vi "test_Compare Avg Access Speed - Var Dict.vi"() -> ()   [LabVIEW 2015]
uses:
  Test Object/Test Object.lvclass
  Test Object/Test Object.lvclass/Test Object.ctl
  objdict/objdict.lvclass
panel:
  out "Average test duration [ms]":dbl[][](array[numeric]) format="%#.6p"
  # "Access Object"
  # "Access and Read Object"
  # "Access and Modify Object"
  # "Variant dict"
  # "objdict"
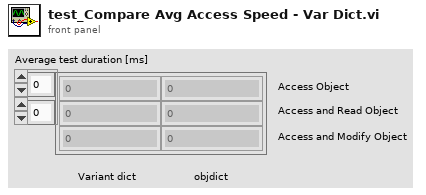
[diagram p1: front panel]
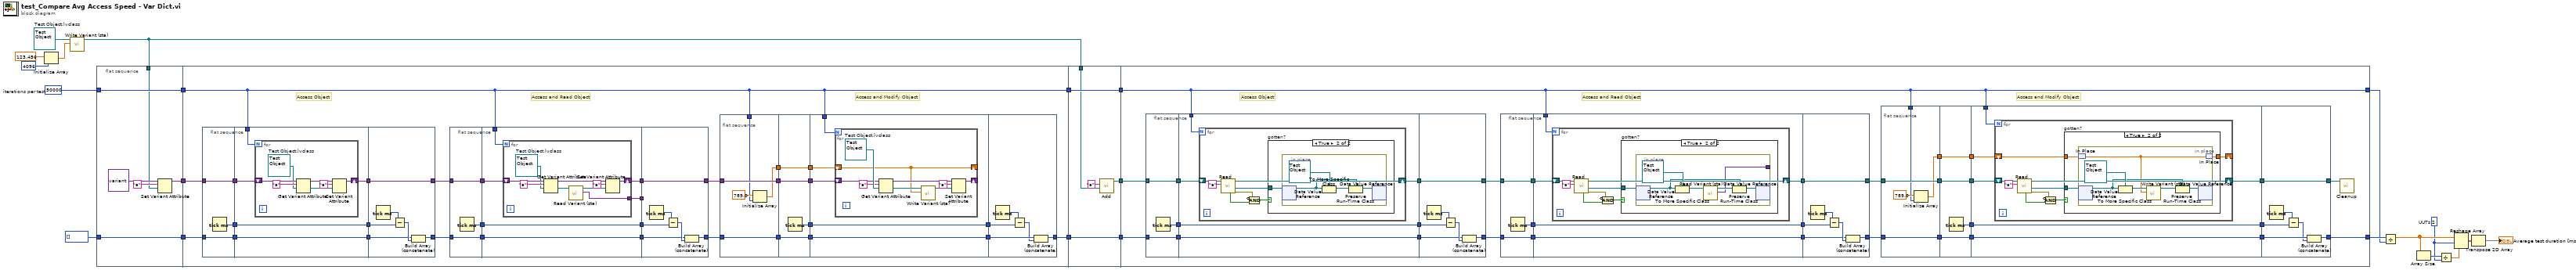
[diagram p0: block diagram]
diagram:
  w2 = 2  # UUTs
  w18 = 50000  # iterations per test
  w23 = refnum<class "Test Object.lvclass"> refnum  # Test Object.lvclass
  n1 = Initialize Array(123.456, 4096) -> (w20:dbl[])
  n2 = call "Write Variant (sta).vi"("Variant"=w20, "Test Object in"=w23) -> ("Test Object out"=w8:refnum<class "Test Object.lvclass">)  [unwired: 9 in]
  n3 = flat-sequence {
    tunnel: w18 -> [w28]
    tunnel: u32[] [] -> [w29]
    tunnel: [w29] -> w13
    tunnel: [w28] -> w12
    tunnel: w8 -> [w25]
    tunnel: [w24] -> w11
    tunnel: w13 -> [w53]
    tunnel: w12 -> [w30]
    tunnel: w11 -> [w42]
    tunnel: [w44] -> w10
    tunnel: [w30] -> w9
    tunnel: w10 -> [w137]
    tunnel: w9 -> [w136]
    tunnel: w8 -> [w135]
    tunnel: [w137] -> w7
    tunnel: [w136] -> w6
    tunnel: [w133] -> w5
    tunnel: [w140] -> w15
    tunnel: [w141] -> w16
    tunnel: w7 -> [w142]
    tunnel: w6 -> [w140]
    tunnel: w5 -> [w143]
    frame #0 {
      n4 = Set Variant Attribute(Variant=variant, name="a", value=w25) -> (Variant out=w24:variant)  [unwired: 1 in, 2 out]
    }
    frame #1 {
      # "Access and Read Object"
      # "Access and Modify Object"
      # "Access Object"
      n5 = flat-sequence {
        tunnel: w42 -> [w114]
        tunnel: [w114] -> w59
        tunnel: [w113] -> w58
        tunnel: w53 -> [w112]
        tunnel: [w112] -> w52
        tunnel: w59 -> [w119]
        tunnel: w58 -> [w118]
        tunnel: [w118] -> w57
        tunnel: w52 -> [w117]
        tunnel: [w117] -> w51
        tunnel: w30 -> [w116]
        tunnel: [w115] -> w43
        tunnel: w57 -> [w132]
        tunnel: w51 -> [w129]
        tunnel: [w128] -> w33
        tunnel: [w127] -> w34
        tunnel: w43 -> [w127]
        frame #0 {
          n6 = Tick Count (ms)() -> (millisecond timer value=w113:u32)
        }
        frame #1 {
          n7 = for {
            N: w116 -> [_]
            shift-right: [w124] -> w115
            shift-left: w119 -> [w126]
            w120 = refnum<class "Test Object.lvclass"> refnum  # Test Object.lvclass
            n8 = Get Variant Attribute(Variant=w126, name="a", default value (empty Variant)=w120) -> (duplicate Variant=w125:variant, value=w122:refnum<class "Test Object.lvclass">)  [unwired: 1 in, 2 out]
            n9 = Set Variant Attribute(Variant=w125, name="a", value=w122) -> (Variant out=w124:variant)  [unwired: 1 in, 2 out]
          }
        }
        frame #2 {
          n10 = Tick Count (ms)() -> (millisecond timer value=w131:u32)
          n11 = Subtract(x=w131, y=w132) -> (x-y=w130:u32)
          n12 = Build Array (concatenate)(w129, w130) -> (w128:u32[])
        }
      }
      n13 = flat-sequence {
        tunnel: w34 -> [w62]
        tunnel: [w62] -> w41
        tunnel: [w61] -> w40
        tunnel: w33 -> [w60]
        tunnel: [w60] -> w39
        tunnel: w41 -> [w68]
        tunnel: w40 -> [w67]
        tunnel: [w67] -> w38
        tunnel: w39 -> [w66]
        tunnel: [w66] -> w37
        tunnel: w30 -> [w65]
        tunnel: [w64] -> w36
        tunnel: [w63] -> w35
        tunnel: w38 -> [w83]
        tunnel: w37 -> [w80]
        tunnel: [w79] -> w31
        tunnel: [w78] -> w32
        tunnel: w36 -> [w78]
        tunnel: w35 -> [_]
        frame #0 {
          n14 = Tick Count (ms)() -> (millisecond timer value=w61:u32)
        }
        frame #1 {
          n15 = for {
            N: w65 -> [_]
            shift-right: [w75] -> w64
            shift-left: w68 -> [w77]
            tunnel: [w69] -> w63
            w71 = refnum<class "Test Object.lvclass"> refnum  # Test Object.lvclass
            n16 = Get Variant Attribute(Variant=w77, name="a", default value (empty Variant)=w71) -> (duplicate Variant=w76:variant, value=w73:refnum<class "Test Object.lvclass">)  [unwired: 1 in, 2 out]
            n17 = call "Read Variant (sta).vi"("Test Object in"=w73) -> ("Variant"=w69:variant, "Test Object out"=w70:refnum<class "Test Object.lvclass">)  [unwired: 9 in]
            n18 = Set Variant Attribute(Variant=w76, name="a", value=w70) -> (Variant out=w75:variant)  [unwired: 1 in, 2 out]
          }
        }
        frame #2 {
          n19 = Tick Count (ms)() -> (millisecond timer value=w82:u32)
          n20 = Subtract(x=w82, y=w83) -> (x-y=w81:u32)
          n21 = Build Array (concatenate)(w80, w81) -> (w79:u32[])
        }
      }
      n22 = flat-sequence {
        tunnel: w31 -> [w87]
        tunnel: w32 -> [w88]
        tunnel: [w88] -> w48
        tunnel: [w87] -> w47
        tunnel: [w85] -> w45
        tunnel: w30 -> [w84]
        tunnel: [w92] -> w56
        tunnel: [w91] -> w55
        tunnel: [w90] -> w50
        tunnel: w48 -> [w92]
        tunnel: w47 -> [w90]
        tunnel: [w89] -> w46
        tunnel: w45 -> [w89]
        tunnel: w56 -> [w97]
        tunnel: w55 -> [w96]
        tunnel: [w96] -> w54
        tunnel: w50 -> [w95]
        tunnel: [w95] -> w49
        tunnel: w30 -> [w94]
        tunnel: w46 -> [w93]
        tunnel: w54 -> [w111]
        tunnel: w49 -> [w109]
        tunnel: [w107] -> w44
        frame #0 {
          n23 = Initialize Array(789.0, w84) -> (w85:dbl[])
        }
        frame #1 {
          n24 = Tick Count (ms)() -> (millisecond timer value=w91:u32)
        }
        frame #2 {
          n25 = for {
            N: w94 -> [_]
            shift-right: [w100] -> _
            shift-left: w97 -> [w101]
            shift-right: [w98] -> _
            shift-left: w93 -> [w98]
            w106 = refnum<class "Test Object.lvclass"> refnum  # Test Object.lvclass
            n26 = Get Variant Attribute(Variant=w101, name="a", default value (empty Variant)=w106) -> (duplicate Variant=w102:variant, value=w105:refnum<class "Test Object.lvclass">)  [unwired: 1 in, 2 out]
            n27 = call "Write Variant (sta).vi"("Variant"=w98, "Test Object in"=w105) -> ("Test Object out"=w99:refnum<class "Test Object.lvclass">)  [unwired: 9 in]
            n28 = Set Variant Attribute(Variant=w102, name="a", value=w99) -> (Variant out=w100:variant)  [unwired: 1 in, 2 out]
          }
        }
        frame #3 {
          n29 = Tick Count (ms)() -> (millisecond timer value=w110:u32)
          n30 = Subtract(x=w110, y=w111) -> (x-y=w108:u32)
          n31 = Build Array (concatenate)(w109, w108) -> (w107:u32[])
        }
      }
    }
    frame #2 {
      n32 = call "Add.vi"("LabVIEW Object"=w135, "key"="a") -> ("Object Dictionary out"=w133:refnum<class "objdict.lvclass">)  [unwired: 8 in, 1 out]
    }
    frame #3 {
      # "Access and Read Object"
      # "Access and Modify Object"
      # "Access Object"
      n33 = flat-sequence {
        tunnel: w143 -> [w239]
        tunnel: [w239] -> w168
        tunnel: [w238] -> w167
        tunnel: w142 -> [w237]
        tunnel: [w237] -> w166
        tunnel: w168 -> [w244]
        tunnel: w167 -> [w243]
        tunnel: [w243] -> w165
        tunnel: w166 -> [w242]
        tunnel: [w242] -> w164
        tunnel: w140 -> [w241]
        tunnel: [w240] -> w163
        tunnel: w165 -> [w262]
        tunnel: w164 -> [w259]
        tunnel: [w258] -> w146
        tunnel: [w257] -> w147
        tunnel: w163 -> [w257]
        frame #0 {
          n34 = Tick Count (ms)() -> (millisecond timer value=w238:u32)
        }
        frame #1 {
          n35 = for {
            N: w241 -> [_]
            shift-right: [w246] -> w240
            shift-left: w244 -> [w251]
            n36 = call "Read.vi"("key"="a", "Object Dictionary in"=w251) -> ("error out"=w247:errorcluster, "Object ref"=w248:refnum<data-value>, "Object Dictionary out"=w246:refnum<class "objdict.lvclass">, "found"=w245:bool)  [unwired: 6 in]
            n37 = Compound Arithmetic op=AND(invert w247, w245) -> (w249:bool)
            n38 = case "gotten?" shown="True" w249 {
              tunnel: w248 -> [_ w252]
              frame False {
              }
              frame True {
                n39 = in-place {
                  n40 = in-place-dvr #1(w252) -> (w255:refnum<class>)  [unwired: 1 out]
                  n41 = To More Specific Class(target class=refnum<class "Test Object.lvclass"> refnum ("Test Object.lvclass"), reference=w255) -> (specific class reference=w253:refnum<class "Test Object.lvclass">)  [unwired: 1 in, 1 out]
                  n42 = Preserve Run-Time Class(object in=w253, 2:w255) -> (object out=w254:refnum<class>)  [unwired: 1 in, 1 out]
                  n43 = in-place-dvr #1(w254) -> ()  [unwired: 2 out]
                }
              }
            }
          }
        }
        frame #2 {
          n44 = Tick Count (ms)() -> (millisecond timer value=w261:u32)
          n45 = Subtract(x=w261, y=w262) -> (x-y=w260:u32)
          n46 = Build Array (concatenate)(w259, w260) -> (w258:u32[])
        }
      }
      n47 = flat-sequence {
        tunnel: w147 -> [w171]
        tunnel: [w171] -> w153
        tunnel: [w170] -> w152
        tunnel: w146 -> [w169]
        tunnel: [w169] -> w151
        tunnel: w153 -> [w174]
        tunnel: w152 -> [w176]
        tunnel: [w176] -> w150
        tunnel: w151 -> [w175]
        tunnel: [w175] -> w149
        tunnel: w140 -> [w173]
        tunnel: [w172] -> w148
        tunnel: w150 -> [w196]
        tunnel: w149 -> [w193]
        tunnel: [w192] -> w144
        tunnel: [w191] -> w145
        tunnel: w148 -> [w191]
        frame #0 {
          n48 = Tick Count (ms)() -> (millisecond timer value=w170:u32)
        }
        frame #1 {
          n49 = for {
            N: w173 -> [_]
            shift-right: [w178] -> w172
            shift-left: w174 -> [w183]
            n50 = call "Read.vi"("key"="a", "Object Dictionary in"=w183) -> ("error out"=w179:errorcluster, "Object ref"=w180:refnum<data-value>, "Object Dictionary out"=w178:refnum<class "objdict.lvclass">, "found"=w177:bool)  [unwired: 6 in]
            n51 = Compound Arithmetic op=AND(invert w179, w177) -> (w181:bool)
            n52 = case "gotten?" shown="True" w181 {
              tunnel: w180 -> [_ w184]
              frame False {
              }
              frame True {
                n53 = in-place {
                  in-place-border: [w185] -> _
                  n54 = in-place-dvr #2(w184) -> (w189:refnum<class>)  [unwired: 1 out]
                  n55 = To More Specific Class(target class=refnum<class "Test Object.lvclass"> refnum ("Test Object.lvclass"), reference=w189) -> (specific class reference=w187:refnum<class "Test Object.lvclass">)  [unwired: 1 in, 1 out]
                  n56 = call "Read Variant (sta).vi"("Test Object in"=w187) -> ("Variant"=w185:variant, "Test Object out"=w186:refnum<class "Test Object.lvclass">)  [unwired: 9 in]
                  n57 = Preserve Run-Time Class(object in=w186, 2:w189) -> (object out=w188:refnum<class>)  [unwired: 1 in, 1 out]
                  n58 = in-place-dvr #2(w188) -> ()  [unwired: 2 out]
                }
              }
            }
          }
        }
        frame #2 {
          n59 = Tick Count (ms)() -> (millisecond timer value=w195:u32)
          n60 = Subtract(x=w195, y=w196) -> (x-y=w194:u32)
          n61 = Build Array (concatenate)(w193, w194) -> (w192:u32[])
        }
      }
      n62 = flat-sequence {
        tunnel: w144 -> [w200]
        tunnel: w145 -> [w201]
        tunnel: [w201] -> w162
        tunnel: [w200] -> w161
        tunnel: [w198] -> w160
        tunnel: w140 -> [w197]
        tunnel: [w205] -> w159
        tunnel: [w204] -> w158
        tunnel: [w203] -> w157
        tunnel: w162 -> [w205]
        tunnel: w161 -> [w203]
        tunnel: [w202] -> w156
        tunnel: w160 -> [w202]
        tunnel: w159 -> [w208]
        tunnel: w158 -> [w211]
        tunnel: [w211] -> w155
        tunnel: w157 -> [w210]
        tunnel: [w210] -> w154
        tunnel: w140 -> [w209]
        tunnel: w156 -> [w207]
        tunnel: [w206] -> w139
        tunnel: w155 -> [w236]
        tunnel: w154 -> [w234]
        tunnel: [w232] -> w141
        tunnel: w139 -> [w231]
        tunnel: [w231] -> w138
        frame #0 {
          n63 = Initialize Array(789.0, w197) -> (w198:dbl[])
        }
        frame #1 {
          n64 = Tick Count (ms)() -> (millisecond timer value=w204:u32)
        }
        frame #2 {
          n65 = for {
            N: w209 -> [_]
            shift-right: [w215] -> w206
            shift-left: w208 -> [w220]
            shift-right: [w213] -> _
            shift-left: w207 -> [w214]
            n66 = call "Read.vi"("key"="a", "Object Dictionary in"=w220) -> ("error out"=w216:errorcluster, "Object ref"=w217:refnum<data-value>, "Object Dictionary out"=w215:refnum<class "objdict.lvclass">, "found"=w212:bool)  [unwired: 6 in]
            n67 = Compound Arithmetic op=AND(invert w216, w212) -> (w218:bool)
            n68 = case "gotten?" shown="True" w218 {
              tunnel: w217 -> [_ w224]
              tunnel: w214 -> [w221 w223]
              tunnel: [w221 w222] -> w213
              frame False {
              }
              frame True {
                n69 = in-place {
                  n70 = in-place-match #3(w223) -> (w225:dbl[])
                  n71 = in-place-dvr #4(w224) -> (w229:refnum<class>)  [unwired: 1 out]
                  n72 = To More Specific Class(target class=refnum<class "Test Object.lvclass"> refnum ("Test Object.lvclass"), reference=w229) -> (specific class reference=w227:refnum<class "Test Object.lvclass">)  [unwired: 1 in, 1 out]
                  n73 = call "Write Variant (sta).vi"("Variant"=w225, "Test Object in"=w227) -> ("Test Object out"=w226:refnum<class "Test Object.lvclass">)  [unwired: 9 in]
                  n74 = Preserve Run-Time Class(object in=w226, 2:w229) -> (object out=w228:refnum<class>)  [unwired: 1 in, 1 out]
                  n75 = in-place-dvr #4(w228) -> ()  [unwired: 2 out]
                  n76 = in-place-match #3(w225) -> (w222:dbl[])
                }
              }
            }
          }
        }
        frame #3 {
          n77 = Tick Count (ms)() -> (millisecond timer value=w235:u32)
          n78 = Subtract(x=w235, y=w236) -> (x-y=w233:u32)
          n79 = Build Array (concatenate)(w234, w233) -> (w232:u32[])
        }
      }
      n80 = call "Cleanup.vi"("Object Dictionary"=w138) -> ()  [unwired: 10 in, 1 out]
    }
  }
  n81 = Divide(x=w16, y=w15) -> (x/y=w17:dbl[])
  n82 = Array Size(array=w17) -> (size(s)=w3:i32)
  n83 = Divide(x=w3, y=w2) -> (x/y=w1:dbl)
  n84 = Reshape Array(w17, w2, w1) -> (w4:dbl[][])
  n85 = Transpose 2D Array(2D array=w4) -> (transposed array=→"Average test duration [ms]":dbl[][])
